vi "PXI-Check for DAQ error.vi"(11 "error in (no error)":errorcluster) -> (15 "error out":errorcluster)   [LabVIEW 2020]
uses:
  DAQ Engine VIs/PXI Globals.vi
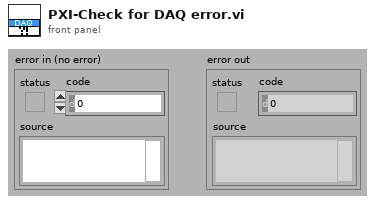
[diagram p1: front panel]
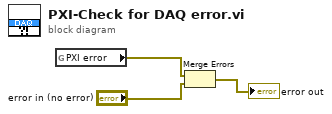
[diagram p0: block diagram]
diagram:
  n1 = global read "PXI Globals.vi" "PXI error"() -> (w3:errorcluster)
  n2 = Merge Errors(w3, "error in (no error)") -> (→"error out":errorcluster)
